vi "Laser_Setup_v1_v19.vi"() -> ()   [LabVIEW 2019]
uses:
  Agilent E363X Series/Agilent E363X Series.lvlib
  SiPM_Tests_Global_Var.vi
  <vilib>/Utility/error.llb/DialogType.ctl
  <vilib>/Instr/_visa.llb/VISA Configure Serial Port (Instr).vi
panel:
  in  "Read Temperature":bool
  out "External Temperature":dbl format="%.2f"
  in  "Boolean":bool
  in  "width":u16=500
  in  "unit":u16(ring) items=["nsec", "usec", "msec"]
  in  "Duty Cycle (%)":u16=50
  out "Pulser ON":bool
  out "Biass ON":bool
  out "Power On":bool
  in  "Waveform":i16(slide)=1 scale=0.0..4.0
  in  "SetPulser":bool
  in  "Enable Bias 3":bool caption="Complementary"
  in  "Enable Bias 2":bool=TRUE caption="Enable Output"
  in  "HP8116A":refnum<visa-resource-name>="GPIB0::16::INSTR" caption="Function Generator HP8116A"
  in  "Trigger mode":i16(slide)=1 scale=0.0..2.0 scale format="%.2f"
  in  "Frequency":ext=3.0
  in  "Unit":u16(ring)=2 items=["mHz", "Hz", "KHz", "MHz"]
  in  "Amplitude (V)":ext=0.2 format="%.3f"
  in  "Offset (V)":ext format="%.3f"
  in  "Voltage Level (V) 3":dbl=-28.0 caption="SiPM Bias (V)" min=-40.0 max=40.0 step=0.1 format="%.3g"
  in  "Enable Bias":bool=TRUE caption="Enable Output"
  in  "Set Bias":bool
  in  "Set Voltage":bool
  in  "Read Voltage":bool
  out "Actual (V) Level":dbl format="%.3g"
  out "Actual (A) Level":dbl format="%.3g"
  out "Actual (V) Level (2)":dbl caption="Actual (V) Level" format="%.3g"
  out "Actual (A) Level (2)":dbl caption="Actual (A) Level" format="%.3g"
  out "Actual (V) Level 2":dbl caption="Actual (V) Level" format="%.3g"
  out "Actual (A) Level 2":dbl caption="Actual (A) Level" format="%.3g"
  in  "Voltage Level (V)":dbl min=0.0 max=25.0 step=0.001 format="%.3g"
  in  "Enable Output":bool=TRUE
  in  "Voltage Level (V) (2)":dbl min=-25.0 max=0.0 step=0.001 format="%.3g"
  in  "Current Limit (A)":dbl=1.0 format="%.3g"
  in  "Current Limit (A) 2":dbl=1.0 caption="Current Limit (A)" format="%.3g"
  in  "Voltage Level (V) 2":dbl=1.8 caption="Voltage Level (V)" min=0.0 max=25.0 step=0.001 format="%.3g"
  in  "Current Limit (A) 3":dbl=1.0 caption="Current Limit (A)" format="%.3g"
  in  "Stop VI":bool
  in  "Default Settings":bool
  in  "Serial Settings":T1={"VISA resource name"="COM3", "baud rate"=9600, "data bits"=8, "parity"=enum."None", "stop bits"=10, "flow control"=0} {"flow control" items=["None"=0, "XON/XOFF"=1, "RTS/CTS"=2, "DTR/DSR"=4]; "stop bits" items=["1.0"=10, "1.5"=15, "2.0"=20]; "data bits" min=5 max=8 step=1}
  out "Serial Monitor":string
  in  "Motor Home":bool
  in  "Step Size (mm)":u32
  in  "X Back":bool
  in  "X forward":bool
  in  "Y back":bool
  in  "Y forward":bool
  # "NCSR  DEMOKRITOS\nInstitute of Nuclear and Particle Physics\nDetectors Instrumentation Laboratory"
  # "Laser Setup System Configuration"
  # "Power Supply Agilent E3631A"
  # "Function Generator HP8116A"
  # "Keithley 6517A"
  # "Stepper Motor"
  # "Arduino Configuration"
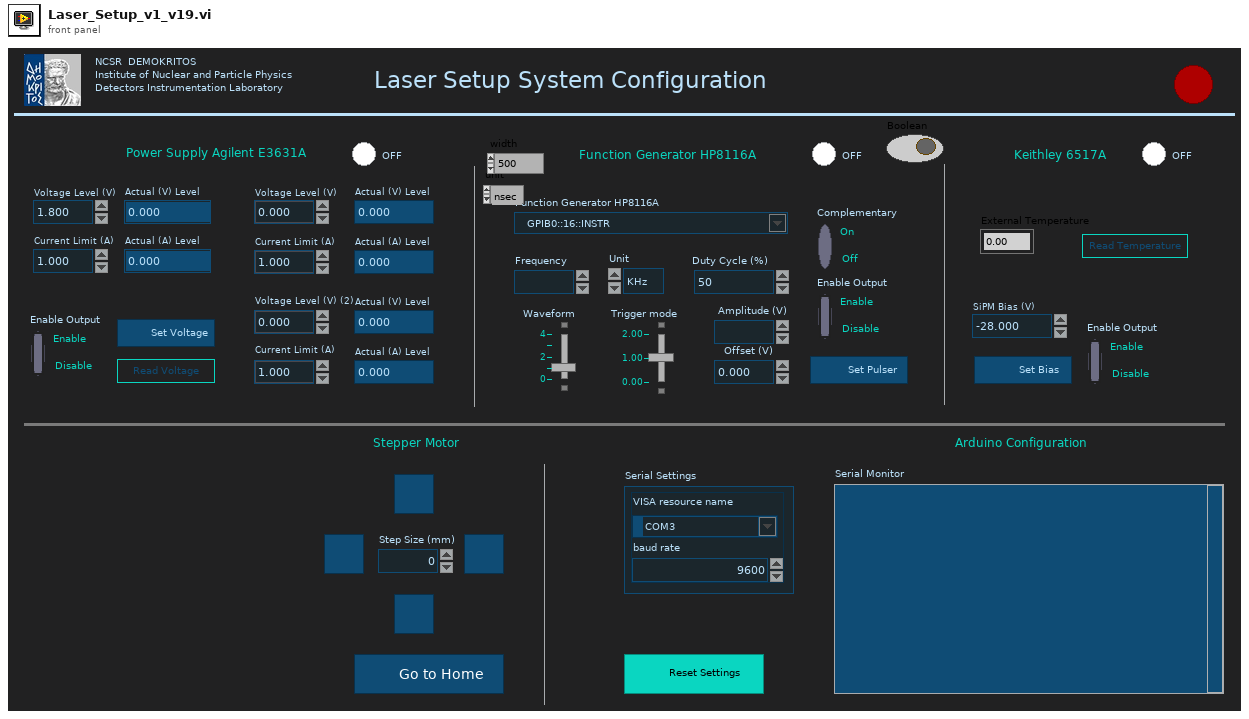
[diagram p1: front panel]
types:
  T1 = cluster{"VISA resource name":refnum<visa-resource-name>, "baud rate":u32, "data bits":u16, "parity":enum16{"None", "Odd", "Even", "Mark", "Space"}, "stop bits":u16, "flow control":u16}
  T2 = typedef "DialogType.ctl" = u16
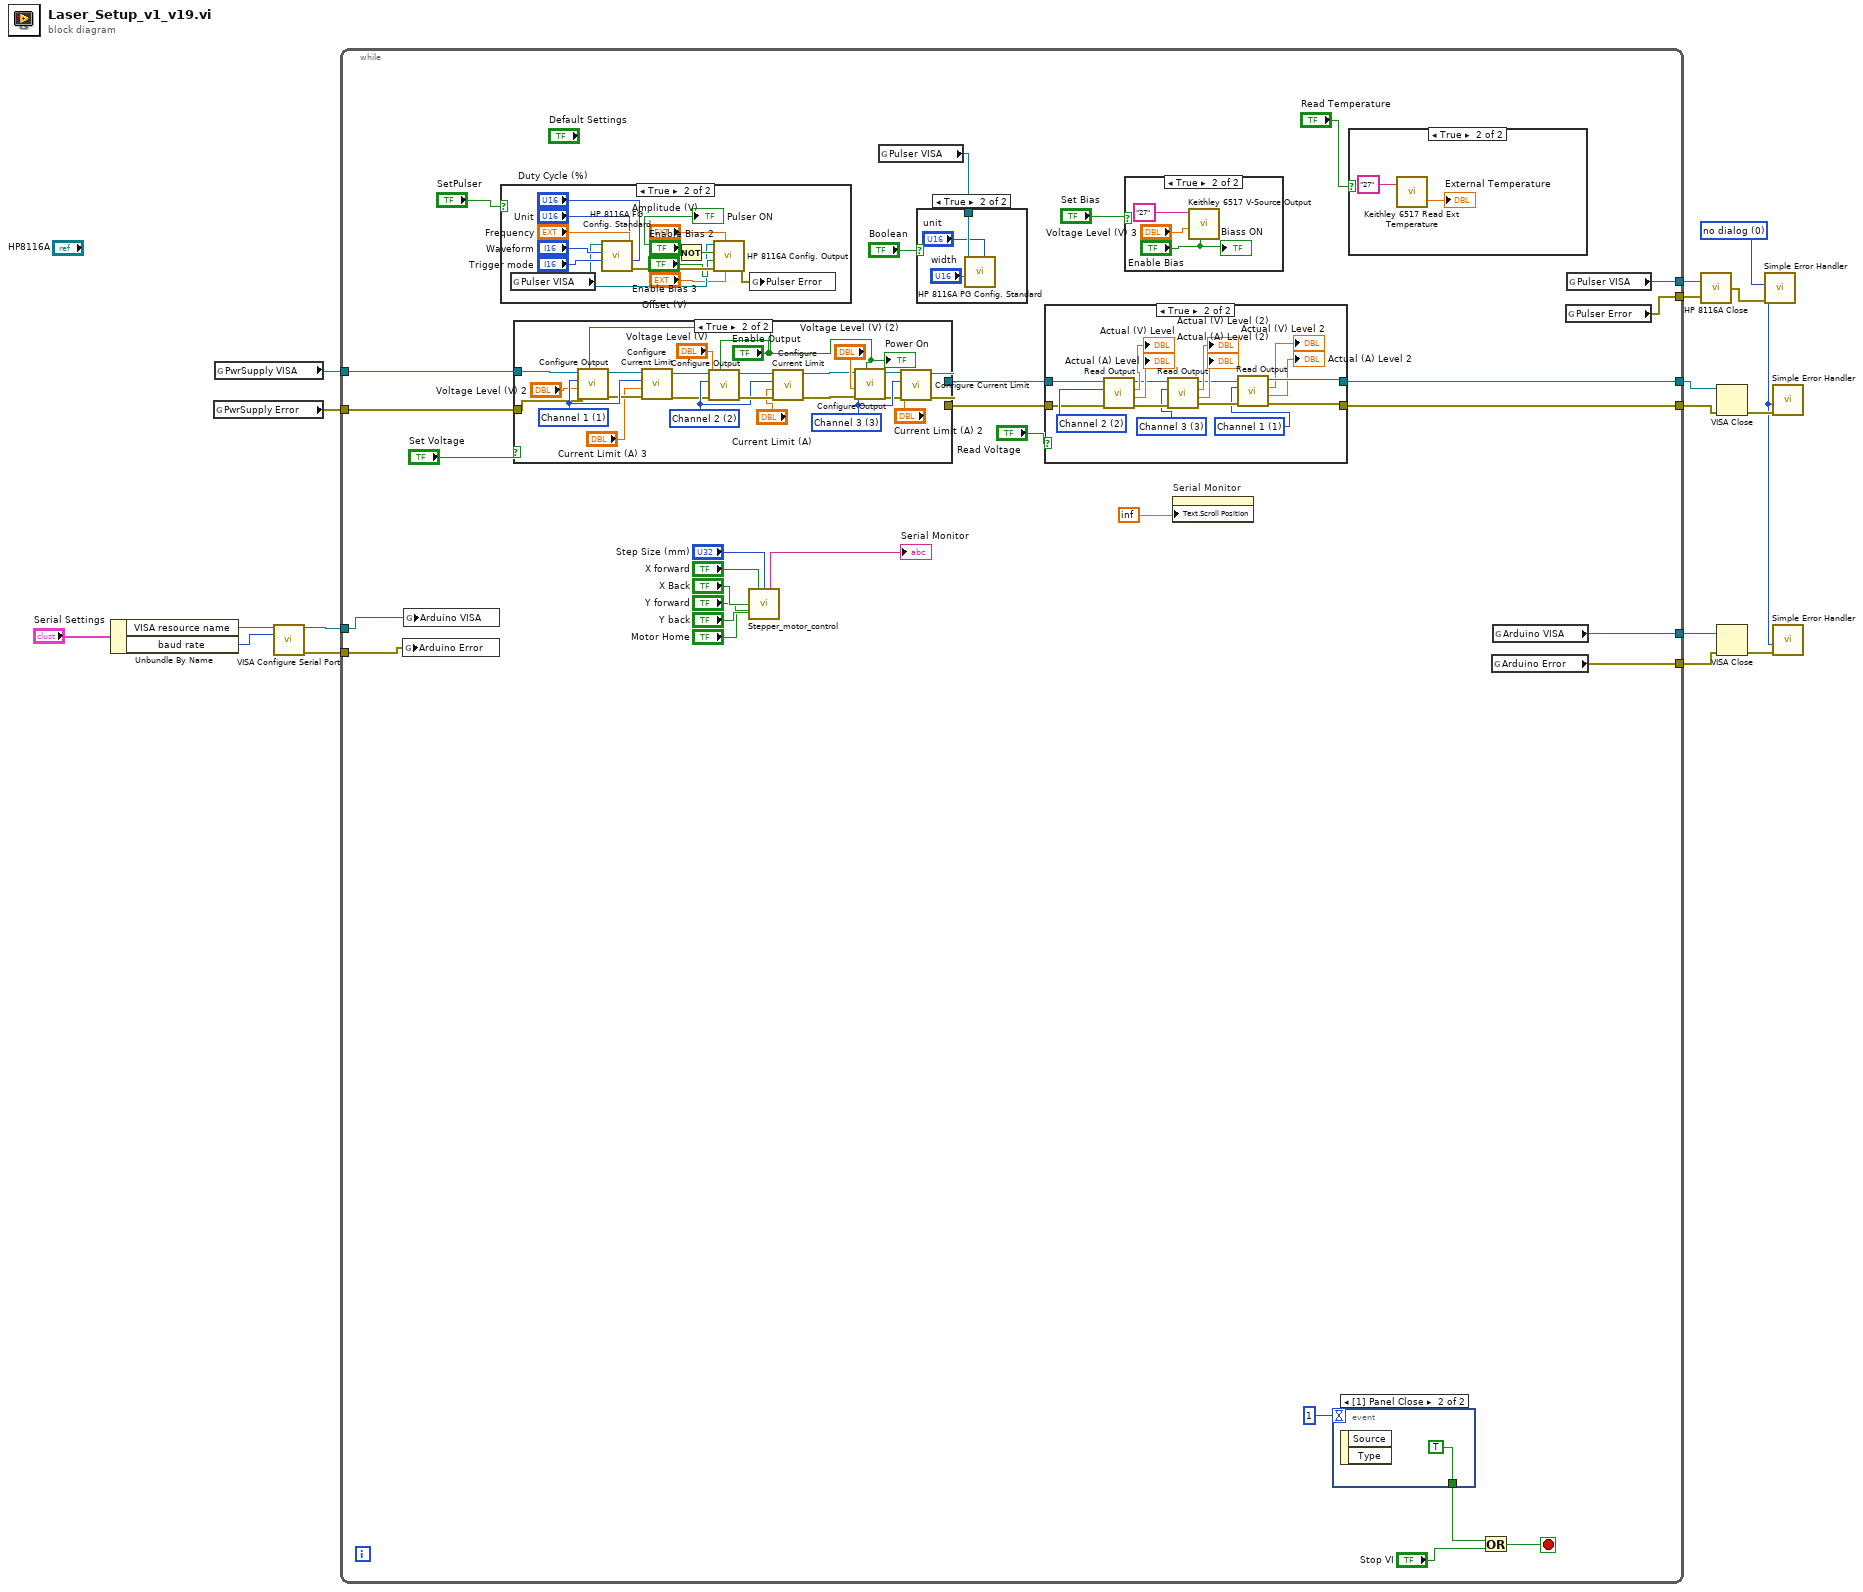
[diagram p0: block diagram]
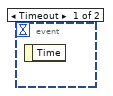
[diagram p8: hidden frame]
diagram:
  w3 = T2 0 items=["no dialog", "OK message", "continue or stop message", "OK message + warnings", "continue/stop + warnings"] ("type of dialog (OK msg:1)")
  n1 = Unbundle By Name("Serial Settings") -> ("VISA resource name"=w13:refnum<visa-resource-name>, "baud rate"=w14:u32)
  n2 = global read "SiPM_Tests_Global_Var.vi" "PwrSupply Error"() -> (w5:errorcluster)
  n3 = global read "SiPM_Tests_Global_Var.vi" "PwrSupply VISA"() -> (w6:refnum<visa-resource-name>)
  n4 = call-poly "VISA Configure Serial Port"("VISA resource name"=w13, "baud rate (9600)"=w14) -> ("VISA resource name out"=w17:refnum<visa-resource-name>, "error out"=w16:errorcluster)  [unwired: 7 in, 5 out]
  n5 = while {
    tunnel: w17 -> [w20]
    tunnel: w16 -> [w19]
    tunnel: [w35] -> w10
    tunnel: [w34] -> w9
    tunnel: [w31] -> w8
    tunnel: [w30] -> w7
    tunnel: w6 -> [w29]
    tunnel: w5 -> [w28]
    tunnel: [w22] -> w2
    tunnel: [w21] -> w1
    stop <- w42 stop-if-true
    n6 = global write "SiPM_Tests_Global_Var.vi" "Arduino Error"(w19) -> ()
    n7 = global write "SiPM_Tests_Global_Var.vi" "Arduino VISA"(w20) -> ()
    n8 = case shown="True" "SetPulser" {
      frame False {
      }
      frame True {
        n9 = global read "SiPM_Tests_Global_Var.vi" "Pulser VISA"() -> (w58:refnum<visa-resource-name>)
        n10 = call "HP 8116A FG Config. Standard.vi"("duty cycle (50 %)"="Duty Cycle (%)", "unit (Hz)"="Unit", "frequency(1000)"="Frequency", "trigger mode (2:normal)"="Trigger mode", "waveform(1:sine)"="Waveform", "VISA session"=w58) -> ("error out"=w63:errorcluster)  [unwired: 4 in]
        n11 = Not(x="Enable Bias 2") -> (.not. x?=w62:bool)
        n12 = call "HP 8116A Config. Output.vi"("offset (V)"="Offset (V)", "amplitude (V)"="Amplitude (V)", "error in (no error)"=w63, "compl\n(F:off)"="Enable Bias 3", "disable\noutput\n(F:off)"=w62, "VISA session"=w58) -> ("error out"=w57:errorcluster)  [unwired: 5 in]
        n13 = global write "SiPM_Tests_Global_Var.vi" "Pulser Error"(w57) -> ()
        "Pulser ON" <- "Enable Bias 2"
      }
    }
    n14 = case shown="True" "Set Voltage" {
      tunnel: [w90 w103] -> w37
      tunnel: [w89 w102] -> w38
      tunnel: w29 -> [w90 w92]
      tunnel: w28 -> [w89 w91]
      frame False {
      }
      frame True {
        w101 = 1 items=["Channel 1"=1, "Channel 2"=2, "Channel 3"=3] ("Channel (1: Channel 1)")
        w106 = 3 items=["Channel 1"=1, "Channel 2"=2, "Channel 3"=3] ("Channel (1: Channel 1)")
        w99 = 2 items=["Channel 1"=1, "Channel 2"=2, "Channel 3"=3] ("Channel (1: Channel 1)")
        n15 = call "Configure Output.vi"("Enable Output (T: Enable)"="Enable Output", "error in (no error)"=w91, "Voltage Level (0.0 V)"="Voltage Level (V) 2", "Channel (1: Channel 1)"=w101, "VISA resource name"=w92) -> ("error out"=w100:errorcluster, "VISA resource name out"=w98:refnum<visa-resource-name>)  [unwired: 5 in]
        n16 = call "Configure Current Limit.vi"("error in (no error)"=w100, "Current Limit (0.0 A)"="Current Limit (A) 3", "Channel (1: Channel 1)"=w101, "VISA resource name"=w98) -> ("error out"=w96:errorcluster, "VISA resource name out"=w97:refnum<visa-resource-name>)  [unwired: 6 in]
        n17 = call "Configure Output.vi"("Enable Output (T: Enable)"="Enable Output", "error in (no error)"=w96, "Voltage Level (0.0 V)"="Voltage Level (V)", "Channel (1: Channel 1)"=w99, "VISA resource name"=w97) -> ("error out"=w111:errorcluster, "VISA resource name out"=w112:refnum<visa-resource-name>)  [unwired: 5 in]
        n18 = call "Configure Current Limit.vi"("error in (no error)"=w111, "Current Limit (0.0 A)"="Current Limit (A)", "Channel (1: Channel 1)"=w99, "VISA resource name"=w112) -> ("error out"=w108:errorcluster, "VISA resource name out"=w109:refnum<visa-resource-name>)  [unwired: 6 in]
        n19 = call "Configure Output.vi"("Enable Output (T: Enable)"="Enable Output", "error in (no error)"=w108, "Voltage Level (0.0 V)"="Voltage Level (V) (2)", "Channel (1: Channel 1)"=w106, "VISA resource name"=w109) -> ("error out"=w105:errorcluster, "VISA resource name out"=w107:refnum<visa-resource-name>)  [unwired: 5 in]
        n20 = call "Configure Current Limit.vi"("error in (no error)"=w105, "Current Limit (0.0 A)"="Current Limit (A) 2", "Channel (1: Channel 1)"=w106, "VISA resource name"=w107) -> ("error out"=w102:errorcluster, "VISA resource name out"=w103:refnum<visa-resource-name>)  [unwired: 6 in]
        "Power On" <- "Enable Output"
      }
    }
    n21 = call "Stepper_motor_control.vi"("X forward"="X forward", "Step Size (mm)"="Step Size (mm)", "X Back"="X Back", "Y forward"="Y forward", "Y back"="Y back", "Motor Home"="Motor Home") -> ("Serial"=→"Serial Monitor":string)  [unwired: 6 in, 3 out]
    n22 = global read "SiPM_Tests_Global_Var.vi" "Pulser VISA"() -> (w27:refnum<visa-resource-name>)
    n23 = case shown="True" "Boolean" {
      tunnel: w27 -> [_ w53]
      frame False {
      }
      frame True {
        n24 = call "HP 8116A PG Config. Standard.vi"("width"="width", "unit"="unit", "VISA session"=w53) -> ()  [unwired: 7 in, 1 out]
      }
    }
    n25 = case shown="True" "Read Voltage" {
      tunnel: w37 -> [w71 w80]
      tunnel: w38 -> [w70 w79]
      tunnel: [w71 w75] -> w35
      tunnel: [w70 w74] -> w34
      frame False {
      }
      frame True {
        w76 = 1 items=["Channel 1"=1, "Channel 2"=2, "Channel 3"=3] ("Channel (1: Channel 1)")
        w83 = 3 items=["Channel 1"=1, "Channel 2"=2, "Channel 3"=3] ("Channel (1: Channel 1)")
        w88 = 2 items=["Channel 1"=1, "Channel 2"=2, "Channel 3"=3] ("Channel (1: Channel 1)")
        n26 = call "Read Output.vi"("error in (no error)"=w79, "Channel (1: Channel 1)"=w88, "VISA resource name"=w80) -> ("error out"=w84:errorcluster, "Actual Current Level (A)"=→"Actual (A) Level":dbl, "Actual Voltage Level (V)"=→"Actual (V) Level":dbl, "VISA resource name out"=w85:refnum<visa-resource-name>)  [unwired: 5 in]
        n27 = call "Read Output.vi"("error in (no error)"=w84, "Channel (1: Channel 1)"=w83, "VISA resource name"=w85) -> ("error out"=w77:errorcluster, "Actual Current Level (A)"=→"Actual (A) Level (2)":dbl, "Actual Voltage Level (V)"=→"Actual (V) Level (2)":dbl, "VISA resource name out"=w78:refnum<visa-resource-name>)  [unwired: 5 in]
        n28 = call "Read Output.vi"("error in (no error)"=w77, "Channel (1: Channel 1)"=w76, "VISA resource name"=w78) -> ("error out"=w74:errorcluster, "Actual Current Level (A)"=→"Actual (A) Level 2":dbl, "Actual Voltage Level (V)"=→"Actual (V) Level 2":dbl, "VISA resource name out"=w75:refnum<visa-resource-name>)  [unwired: 5 in]
      }
    }
    n29 = case shown="True" "Set Bias" {
      frame False {
      }
      frame True {
        n30 = call "Keithley 6517 V-Source Output.vi"("V-Source Operate"="Enable Bias", "Output Voltage Value"="Voltage Level (V) 3", "GPIB address"="27") -> ()  [unwired: 7 in, 1 out]
        "Biass ON" <- "Enable Bias"
      }
    }
    n31 = property on="Serial Monitor" class="Str"("Text.Scroll Position"=inf) -> ()  [unwired: 2 in, 2 out]
    n32 = event shown="[1] Panel Close" {
      selector: _ -> [_ _]
      dyn-events: _ -> [_ _]
      timeout: 1 -> [_ _]
      tunnel: [_ TRUE] -> w41
      event Timeout {
        n33 = event-data() -> ()  [unwired: 1 in, 1 out]
      }
      event Panel Close {
        n34 = event-data() -> ()  [unwired: 1 in, 2 out]
      }
    }
    n35 = case shown="True" "Read Temperature" {
      frame False {
      }
      frame True {
        n36 = call "Keithley 6517 Read Ext Temperature.vi"("GPIB address"="27") -> ("External Temperature"=→"External Temperature":dbl)  [unwired: 1 in, 1 out]
      }
    }
    n37 = Or(x=w41, y="Stop VI") -> (x .or. y?=w42:bool)
    n38 = global read "SiPM_Tests_Global_Var.vi" "Arduino Error"() -> (w21:errorcluster)
    n39 = global read "SiPM_Tests_Global_Var.vi" "Arduino VISA"() -> (w22:refnum<visa-resource-name>)
    n40 = global read "SiPM_Tests_Global_Var.vi" "Pulser Error"() -> (w30:errorcluster)
    n41 = global read "SiPM_Tests_Global_Var.vi" "Pulser VISA"() -> (w31:refnum<visa-resource-name>)
  }
  n42 = call "HP 8116A Close.vi"("error in (no error)"=w7, "VISA session"=w8) -> ("error out"=w4:errorcluster)
  n43 = VISA Close(VISA resource name=w10, error in (no error)=w9) -> (error out=w11:errorcluster)
  n44 = VISA Close(VISA resource name=w2, error in (no error)=w1) -> (error out=w15:errorcluster)
  n45 = call <vilib>:"Simple Error Handler.vi"("type of dialog (OK msg:1)"=w3, "error in (no error)"=w4) -> ()  [unwired: 8 out]
  n46 = call <vilib>:"Simple Error Handler.vi"("type of dialog (OK msg:1)"=w3, "error in (no error)"=w11) -> ()  [unwired: 8 out]
  n47 = call <vilib>:"Simple Error Handler.vi"("type of dialog (OK msg:1)"=w3, "error in (no error)"=w15) -> ()  [unwired: 8 out]
